vi "OnRefeeChange.vi"(0 "XRef":T11, 1 "IDs":T9, 2 "State In":T1) -> (14 "Reply":T9, 15 "Fatal Error Out":T8, 16 "State Out":T1)   [LabVIEW 2020, in "Parallel Diagram Block.xnode"]
uses:
  Parallel Diagram Block.xnode
  <vilib>/XNodeSupport/XNodeXNodeRef.ctl
  <vilib>/XNodeSupport/XNodeStringArray.ctl
  <vilib>/XNodeSupport/XNodeString.ctl
  State.ctl
  Parallel Block/Type Descriptor.ctl
  Parallel Block/Value Type.ctl
  Parallel Block/Terminal Mode.ctl
  <vilib>/picture/picture.llb/imagedata.ctl
  Parallel Block/IO Selection.ctl
  Parallel Block/Direction.ctl
  <vilib>/XNodeSupport/XNodeErrorCluster.ctl
  <vilib>/XNodeSupport/NI_XNodeSupport.lvlib
  Parallel Block/Parallel Block.lvlib
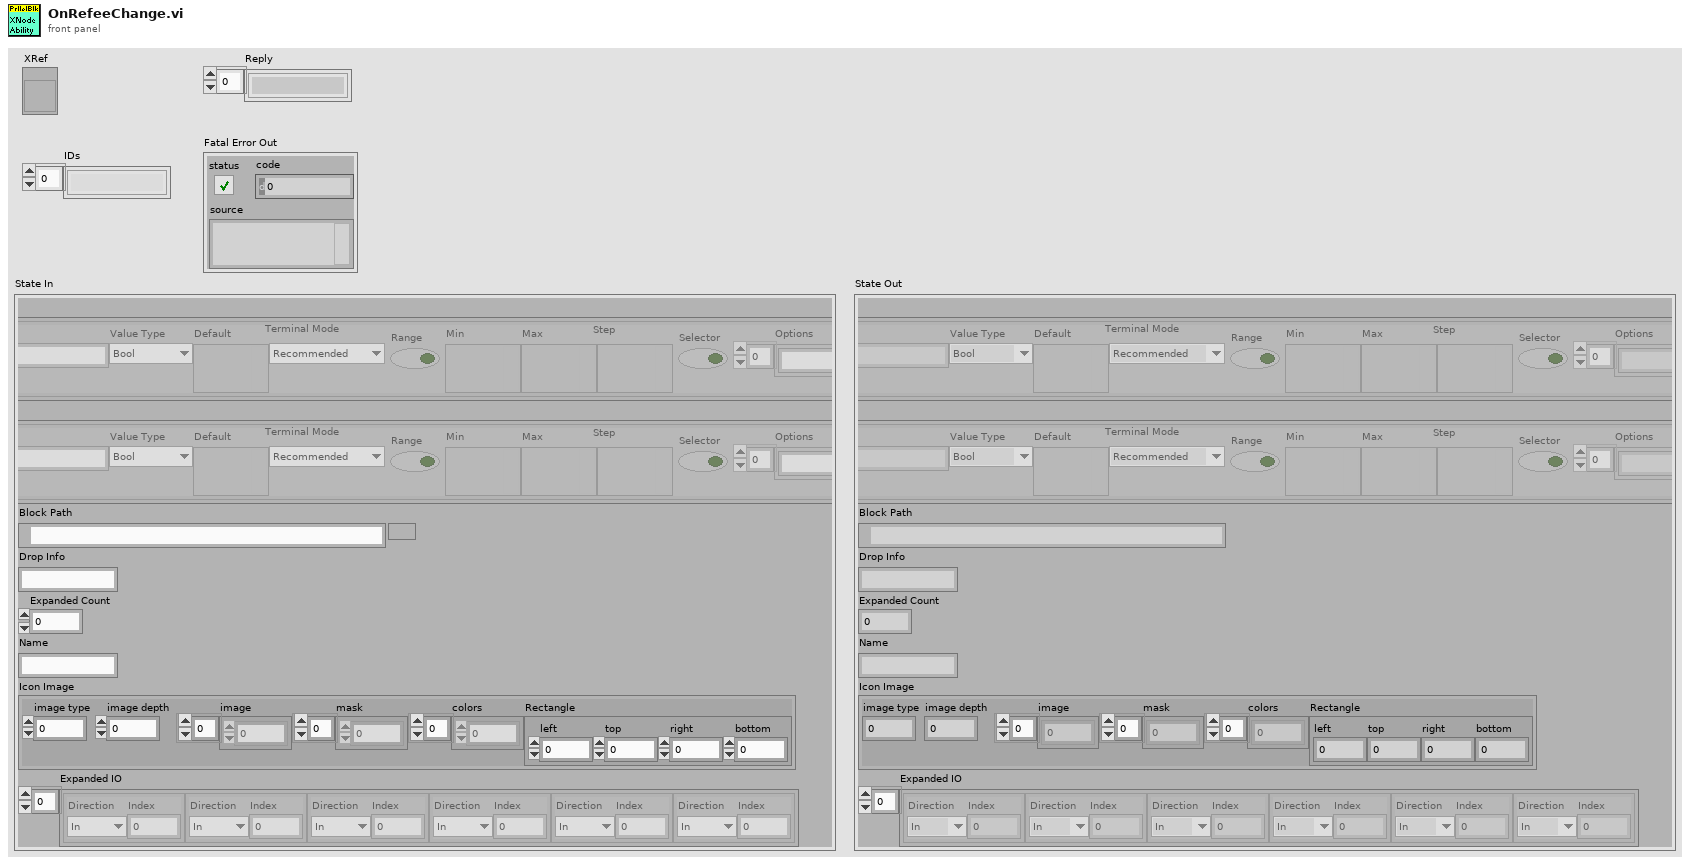
[diagram p1: front panel]
types:
  T1 = typedef "Parallel Diagram Block.xnode/State.ctl" = cluster{"Input Types":T2[], "Output Types":T2[], "Block Path":path, "Drop Info":string, "Expanded Count":i32, "Name":string, "Icon Image":T5, "Expanded IO":T6[]}
  T2 = typedef "Parallel Block.lvlib/Type Descriptor.ctl" = cluster{"Name":string, "Value Type":T3, "Default":variant, "Terminal Mode":T4, "Range":bool, "Min":variant, "Max":variant, "Step":variant, "Selector":bool, "Options":string[]}
  T3 = typedef "Parallel Block.lvlib/Value Type.ctl" = enum16{"Unknown", "Bool", "U8", "U16", "U32", "U64", "I8", "I16", "I32", "I64", "SGL", "DBL", "CSG", "CDB", "CDBWfm", "String", "DBLWfm"}
  T4 = typedef "Parallel Block.lvlib/Terminal Mode.ctl" = enum16{"Recommended", "Required", "None"}
  T5 = typedef "imagedata.ctl" = cluster{"image type":i32, "image depth":i32, "image":u8[], "mask":u8[], "colors":u32[], "Rectangle":cluster{"left":i16, "top":i16, "right":i16, "bottom":i16}}
  T6 = typedef "Parallel Block.lvlib/IO Selection.ctl" = cluster{"Direction":T7, "Index":i32}
  T7 = typedef "Parallel Block.lvlib/Direction.ctl" = enum16{"In", "Out"}
  T8 = typedef "NI_XNodeSupport.lvlib/XNodeErrorCluster.ctl" = errorcluster
  T9 = typedef "NI_XNodeSupport.lvlib/XNodeStringArray.ctl" = T10[]
  T10 = typedef "NI_XNodeSupport.lvlib/XNodeString.ctl" = string
  T11 = typedef "NI_XNodeSupport.lvlib/XNodeXNodeRef.ctl" = refnum<vi>
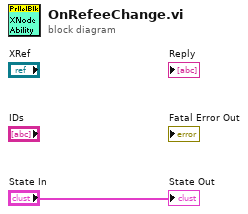
[diagram p0: block diagram]
diagram:
  "State Out" <- "State In"
